vi "mono-config.vi"(8 "error in (no error)":errorcluster, 11 "Monochromator":refnum<vi>) -> (0 "error out":errorcluster)   [LabVIEW 2016]
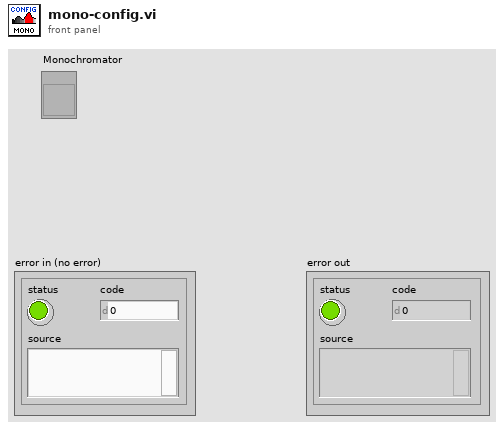
[diagram p1: front panel]
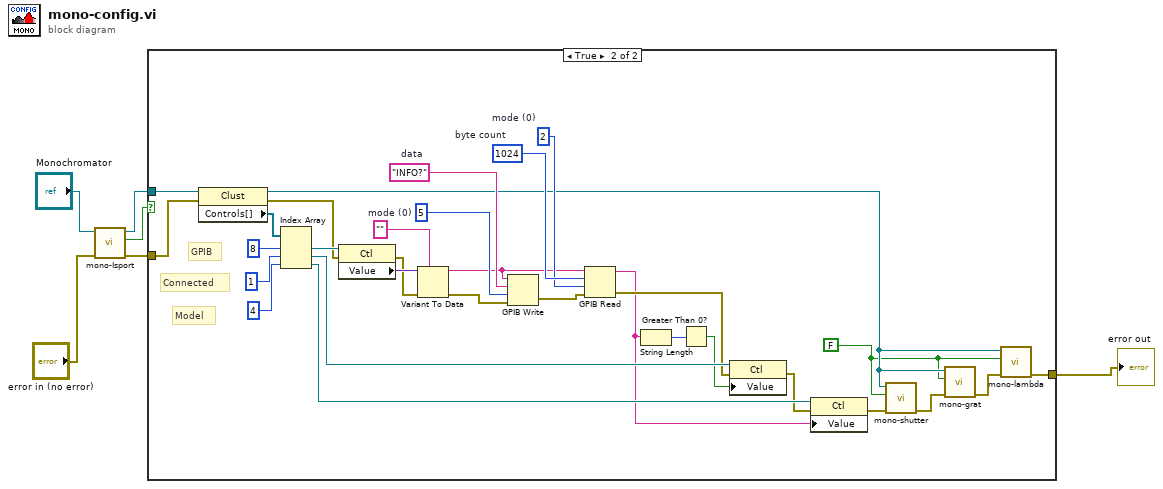
[diagram p0: block diagram]
diagram:
  n1 = call "mono-Isport.vi"("error in (no error)"="error in (no error)", "Monochromator"="Monochromator") -> ("Error Out"=w5:errorcluster, "Boolean"=w3:bool, "Monochromator out"=w4:refnum<vi>)  [unwired: 7 in]
  n2 = case shown="True" w3 {
    tunnel: w5 -> [w7 w28]
    tunnel: [w7 w8] -> w6
    tunnel: w4 -> [_ w31]
    frame False {
    }
    frame True {
      w9 = FALSE ("Set")
      w38 = 1024  # byte count
      w37 = i16 2  # mode (0)
      w36 = "INFO?"  # data
      w35 = i16 5  # mode (0)
      # "Model"
      # "Connected"
      # "GPIB"
      n3 = property class="Clust"(reference=w31, error in=w28) -> (reference out=w10:refnum<vi>, error out=w26:errorcluster, "Controls[]"=w30:refnum<vi>[])
      n4 = Index Array(array=w30, index #1=8 ("index"), index #2=1 ("index"), index #3=4 ("index")) -> (element #1=w27:refnum<vi>, element #2=w18:refnum<vi>, element #3=w14:refnum<vi>)
      n5 = property class="Ctl"(reference=w27, error in=w26) -> (error out=w23:errorcluster, "Value"=w25:variant)  [unwired: 1 out]
      n6 = Variant To Data(error in=w23, type="", Variant=w25) -> (data=w20:string, error out=w22:errorcluster)
      n7 = GPIB Write(0:w20, 1:w36, 2:w35, 3:w22) -> (6:w21:errorcluster)  [unwired: 1 in, 1 out]
      n8 = GPIB Read(0:w20, 1:w38, 2:w37, 3:w21) -> (5:w12:string, 7:w16:errorcluster)  [unwired: 1 in, 1 out]
      n9 = String Length(string=w12) -> (length=w34:i32)
      n10 = Greater Than 0?(x=w34) -> (x > 0?=w17:bool)
      n11 = property class="Ctl"(reference=w18, error in=w16, "Value"=w17) -> (error out=w13:errorcluster)  [unwired: 1 out]
      n12 = property class="Ctl"(reference=w14, error in=w13, "Value"=w12) -> (error out=w11:errorcluster)  [unwired: 1 out]
      n13 = call "mono-shutter.vi"("error in (no error)"=w11, "Set"=w9, "Monochromator"=w10) -> ("error out"=w33:errorcluster)  [unwired: 8 in]
      n14 = call "mono-grat.vi"("Error In"=w33, "Set"=w9, "Mono"=w10) -> ("Error Out"=w32:errorcluster)  [unwired: 8 in]
      n15 = call "mono-lambda.vi"("Error In"=w32, "set"=w9, "Monochromator"=w10) -> ("Error Out"=w8:errorcluster)  [unwired: 8 in]
    }
  }
  "error out" <- w6
